vi "_add to array.vi"(8 "i":errorcluster, 10 "A in":refnum<class "Value.lvclass">[](array[class]), 11 "Value in":refnum<class "Value.lvclass">) -> (0 "error out":errorcluster, 2 "A out":refnum<class "Value.lvclass">[](array[class]), 3 "Value out":refnum<class "Value.lvclass">)   [LabVIEW 2023, in "LabGRAD.lvlib" / "Value.lvclass"]
uses:
  Value.lvclass
  Value.lvclass/Value.ctl
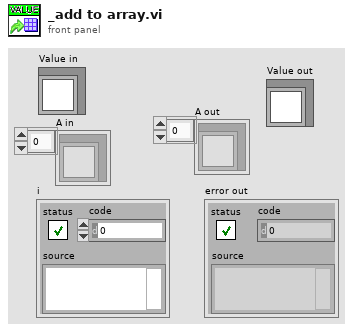
[diagram p1: front panel]
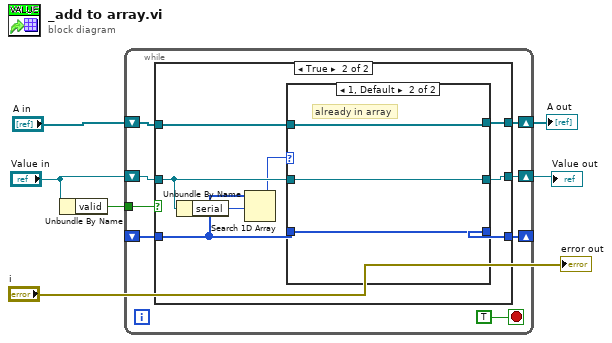
[diagram p0: block diagram]
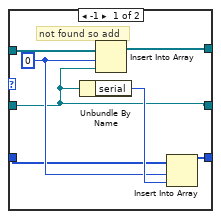
[diagram p3: hidden frame]
diagram:
  n1 = Unbundle By Name("Value in") -> ("valid"=w6:bool)
  n2 = while {
    tunnel: w6 -> [w14]
    shift-right: [w11] -> w3
    shift-left: "A in" -> [w13]
    shift-right: [w10] -> w2
    shift-left: "Value in" -> [w12]
    shift-right: [w8] -> _
    shift-left: _ -> [w7]
    stop <- TRUE stop-if-true
    n3 = case shown="True" w14 {
      tunnel: w13 -> [w17 w25]
      tunnel: w12 -> [w16 w21]
      tunnel: [w17 w24] -> w11
      tunnel: [w16 w22] -> w10
      tunnel: [w15 w23] -> w8
      tunnel: w7 -> [w15 w20]
      frame False {
      }
      frame True {
        n4 = Unbundle By Name(w21) -> ("serial"=w19:u32)
        n5 = Search 1D Array(1D array=w20, element=w19) -> (index of element=w18:i32)  [unwired: 1 in]
        n6 = case shown="1, Default" w18 {
          tunnel: w25 -> [w32 w33]
          tunnel: [w31 w33] -> w24
          tunnel: w21 -> [w26 w35]
          tunnel: [w28 w34] -> w23
          tunnel: w20 -> [w27 w34]
          tunnel: [w26 w35] -> w22
          frame -1 {
            w29 = 0 ("index")
            # "not found so add"
            n7 = Unbundle By Name(w26) -> ("serial"=w30:u32)
            n8 = Insert Into Array(array=w32, index=w29, new element=w26) -> (w31:refnum<class "Value.lvclass">[])
            n9 = Insert Into Array(array=w27, index=w29, new element=w30) -> (w28:u32[])
          }
          frame 1, Default {
            # "already in array"
          }
        }
      }
    }
  }
  "Value out" <- w2
  "A out" <- w3
  "error out" <- "i"
